vi "Read COMM Status.vi"(8 "error in (no error)":errorcluster, 11 "Hardware in":refnum<class "Hardware.lvclass">) -> (0 "error out":errorcluster, 2 "COMM status":bool, 3 "Hardware out":refnum<class "Hardware.lvclass">)   [LabVIEW 2016, in "Hardware.lvlib" / "Hardware.lvclass"]
uses:
  <userlib>/Common Components/Hardware/Abstract Hardware/Hardware.lvclass
  <userlib>/Common Components/Hardware/Abstract Hardware/Hardware.lvclass/Hardware.ctl
  <userlib>/Common Components/Hardware/DevInfo/DevInfo.lvclass/DevInfo.ctl
  <userlib>/Common Components/Hardware/DevInfo/Read Status.vi
  <userlib>/Common Components/Hardware/DevInfo/DevInfo.lvclass
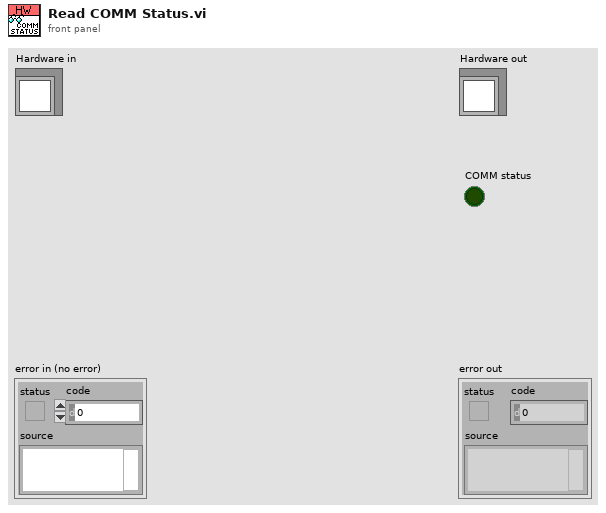
[diagram p1: front panel]
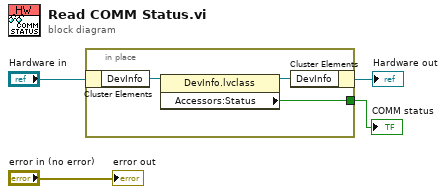
[diagram p0: block diagram]
diagram:
  n1 = in-place {
    in-place-border: [w5] -> w1
    n2 = in-place-cluster #1("Hardware in") -> ("DevInfo"=w7:refnum<class "DevInfo.lvclass">)
    n3 = property class="DevInfo.lvclass"(reference=w7) -> (reference out=w6:refnum<class "DevInfo.lvclass">, "Accessors:Status"=w5:bool)  [unwired: 1 in, 1 out]
    n4 = in-place-cluster #1("DevInfo"=w6) -> (→"Hardware out":refnum<class "Hardware.lvclass">)
  }
  "COMM status" <- w1
  "error out" <- "error in (no error)"
